vi "download file.vi"(8 "error in (no error)":errorcluster, 11 "远端地址":string="/UP/OneStation/V4/一体化微型水质监测站.zip") -> (0 "error out":errorcluster, 3 "local file path":path caption="本地文件路径")   [LabVIEW 2016, in "update.lvlib"]
uses:
  update.lvlib
  <vilib>/WebDAVClient/Advanced/Multi Event/Request Status.ctl
  WebDAV client/WebDAV client.lvclass
  <vilib>/WebDAVClient/NI_WebDAV.lvlib
panel:
  out "request status":T1
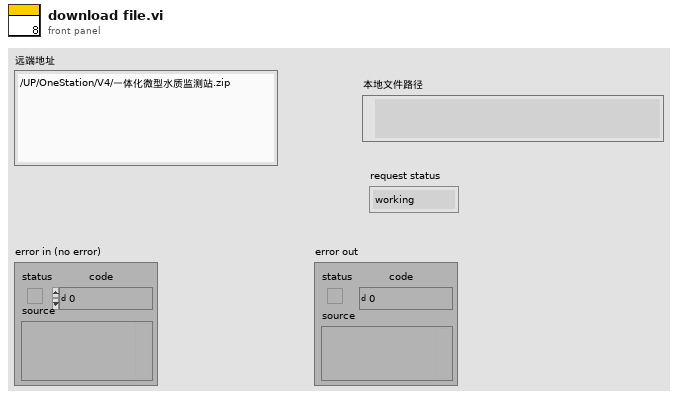
[diagram p1: front panel]
types:
  T1 = typedef "NI_WebDAV.lvlib/Request Status.ctl" = enum16{"working", "complete", "aborted", "timeout", "error"}
  T2 = cluster{"host uri prefix":string, "username":string, "password":string}
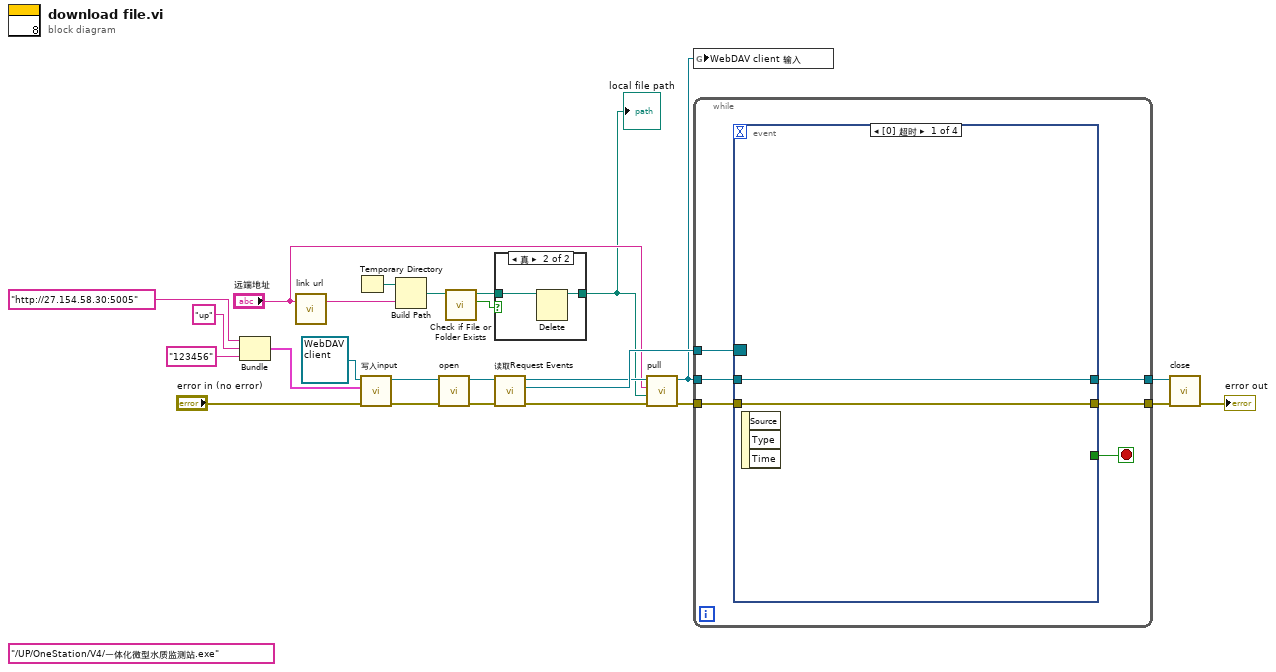
[diagram p0: block diagram]
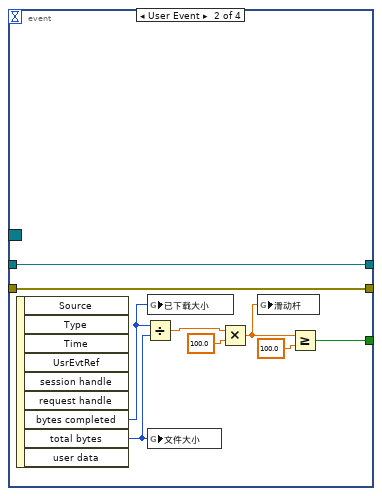
[diagram p3: hidden frame]
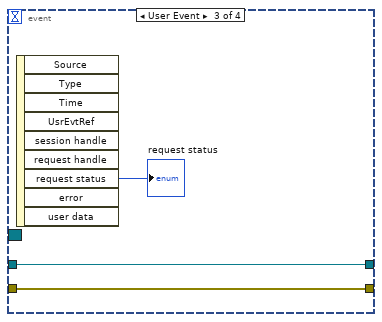
[diagram p4: hidden frame]
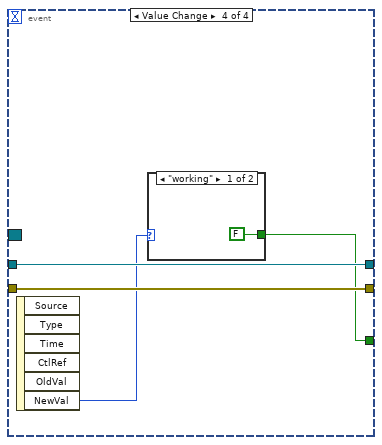
[diagram p5: hidden frame]
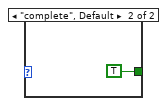
[diagram p6: hidden frame]
diagram:
  (unwired) "/UP/OneStation/V4/一体化微型水质监测站.exe" ("更新包远端地址")
  n1 = Bundle("host uri prefix"="http://27.154.58.30:5005", "username"="up", "password"="123456") -> (w20:T2)  [unwired: 1 in]
  n2 = call "link url.vi"("远端地址"="远端地址") -> ("file name"=w2:string)  [unwired: 17 in, 1 out]
  n3 = Temporary Directory() -> (w6:path)
  n4 = call-dynamic "写入input.vi"("error in (no error)"="error in (no error)", "input"=w20, "WebDAV client输入"=refnum<class "WebDAV client.lvclass"> refnum ("update.lvlib:WebDAV client.lvclass")) -> ("error out"=w19:errorcluster, "WebDAV client输出"=w21:refnum<class "WebDAV client.lvclass">)  [unwired: 7 in]
  n5 = Build Path(base path=w6, name or relative path=w2) -> (appended path=w5:path)
  n6 = call-dynamic "open.vi"("error in (no error)"=w19, "WebDAV client 输入"=w21) -> ("error out"=w18:errorcluster, "WebDAV client 输出"=w17:refnum<class "WebDAV client.lvclass">)  [unwired: 8 in]
  n7 = call <vilib>:"Check if File or Folder Exists.vi"("path"=w5) -> ("file or folder exists?"=w3:bool, "dup path"=w4:path)  [unwired: 8 in, 1 out]
  n8 = case shown="真" w3 {
    tunnel: w4 -> [w26 w28]
    tunnel: [w26 w27] -> w1
    frame False {
    }
    frame True {
      n9 = Delete(path (use dialog)=w28) -> (deleted path=w27:path)  [unwired: 4 in, 2 out]
    }
  }
  "local file path" <- w1
  n10 = call-dynamic "读取Request Events.vi"("error in (no error)"=w18, "WebDAV client输入"=w17) -> ("error out"=w9:errorcluster, "Request Events"=w15:refnum<event-registration>, "WebDAV client输出"=w11:refnum<class "WebDAV client.lvclass">)  [unwired: 7 in]
  n11 = call-dynamic "pull.vi"("error in (no error)"=w9, "local file path"=w1, "更新包远端地址"="远端地址", "WebDAV client 输入"=w11) -> ("error out"=w8:errorcluster, "WebDAV client 输出"=w10:refnum<class "WebDAV client.lvclass">)  [unwired: 6 in]
  n12 = global write "更新全局变量.vi" "WebDAV client 输入"(w10) -> ()
  n13 = while {
    tunnel: w15 -> [w34]
    tunnel: w10 -> [w33]
    tunnel: [w31] -> w14
    tunnel: [w30] -> w13
    tunnel: w8 -> [w29]
    stop <- w32 stop-if-true
    n14 = event shown="[0] 超时" {
      selector: w34 -> [_ _ _ _]
      dyn-events: _ -> [_ _ _ _]
      timeout: _ -> [_ _ _ _]
      tunnel: w33 -> [w36 w38 w47 w52]
      tunnel: [_ w39 _ w49] -> w32
      tunnel: [w36 w38 w47 w52] -> w31
      tunnel: [w35 w37 w46 w51] -> w30
      tunnel: w29 -> [w35 w37 w46 w51]
      event Timeout {
        n15 = event-data() -> ()  [unwired: 1 in, 3 out]
      }
      event User Event {
        n16 = event-data() -> ("bytes completed"=w42:u64, "total bytes"=w43:u64)  [unwired: 1 in, 7 out]
        n17 = Divide(x=w42, y=w43) -> (x/y=w44:dbl)
        n18 = global write "更新全局变量.vi" "已下载大小"(w42) -> ()
        n19 = global write "更新全局变量.vi" "文件大小"(w43) -> ()
        n20 = Multiply(x=w44, y=100.0) -> (x*y=w41:dbl)
        n21 = global write "更新全局变量.vi" "滑动杆"(w41) -> ()
        n22 = Greater Or Equal?(x=w41, y=100.0) -> (x >= y?=w39:bool)
      }
      event User Event {
        n23 = event-data() -> ("request status"=→"request status":T1)  [unwired: 1 in, 8 out]
      }
      event Value Change {
        n24 = event-data() -> ("NewVal"=w50:T1)  [unwired: 1 in, 5 out]
        n25 = case shown="\"working\"" w50 {
          tunnel: [FALSE TRUE] -> w49
          frame "working" {
          }
          frame "complete", Default {
          }
        }
      }
    }
  }
  n26 = call-dynamic "close.vi"("error in (no error)"=w13, "WebDAV client 输入"=w14) -> ("error out"=→"error out":errorcluster)  [unwired: 8 in, 1 out]
